vi "Insert Conditional.vi"(0 "Custom Type Test Executive in":refnum<class "Custom Type Test Executive.lvclass">, 1 "Name":string, 2 "Unique ID":string, 3 "Insertion Index":i32=-1, 4 "Assertion":refnum<class "Assert.lvclass">, 5 "error in (no error)":errorcluster, 6 "Parent ID":string, 7 "Variable X":string, 9 "Variable Y":string, 11 "Passing Executive":string, 13 "Failing Executive":string) -> (12 "Unique ID out":string, 14 "Custom Type Test Executive out":refnum<class "Custom Type Test Executive.lvclass">, 17 "Replaced?":bool, 19 "error out":errorcluster)   [LabVIEW 2017, in "Custom Type Test Executive.lvlib" / "Custom Type Test Executive.lvclass"]
uses:
  <vilib>/gpm_packages/@cs/test-executive/Source/Custom Type Test Executive/Custom Type Test Executive/Custom Type Test Executive.lvclass
  C:/Program Files/National Instruments/LabVIEW 2017/vi.lib/gpm_packages/@cs/test-executive/Source/Test Executive/TestExecutive/Test Executive.lvclass
  <vilib>/gpm_packages/@cs/run-time-assertions/Source/Assert/Assert.lvclass
  <vilib>/gpm_packages/@cs/test-executive/Source/Custom Type Test Executive/Conditional/Conditional.lvclass
  <vilib>/gpm_packages/@cs/data-type-serializer/source/Boolean/Boolean.lvclass/Boolean.ctl
  <vilib>/gpm_packages/@cs/test-executive/Source/Test Executive/TestExecutive/Test Executive.lvclass/Test Executive.ctl
  <vilib>/gpm_packages/@cs/data-type-serializer/source/Assertion/Assertion.lvclass/Assertion.ctl
  <vilib>/gpm_packages/@cs/data-type-serializer/source/String/String.lvclass/String.ctl
  ab7743c9-886f-4ba9-96ef-3eddb2be0c4c.vi
  3e0f2c71-549b-4a67-9684-e53ffa5485a3.vi
  d4ff8dc7-3c29-48bf-87c7-0a5f4c60658c.vi
  dd2f15b4-1a6c-43c8-9979-5ab3f4848fd4.vi
  23726e33-d18f-4018-bfd9-b10ab65a482d.vi
  439cc76c-a804-4d9c-815d-5f0c42b8a7d2.vi
  71fa445d-2d61-434e-a671-de836141d59d.vi
  <vilib>/gpm_packages/@cs/data-type-serializer/source/Assertion/Assertion.lvclass
  <vilib>/gpm_packages/@cs/data-type-serializer/source/String/String.lvclass
  <vilib>/gpm_packages/@cs/data-type-serializer/source/Boolean/Boolean.lvclass
  <vilib>/gpm_packages/@cs/linked-list/Source/Linked List/ILinkedList/ILinked List.lvclass
  <vilib>/gpm_packages/@cs/linked-list/Source/Linked List/Linked List Ref/Linked List Ref.lvclass
  <vilib>/gpm_packages/@cs/test-executive/Source/Test Executive/TestExecutive/Test Executive.lvclass
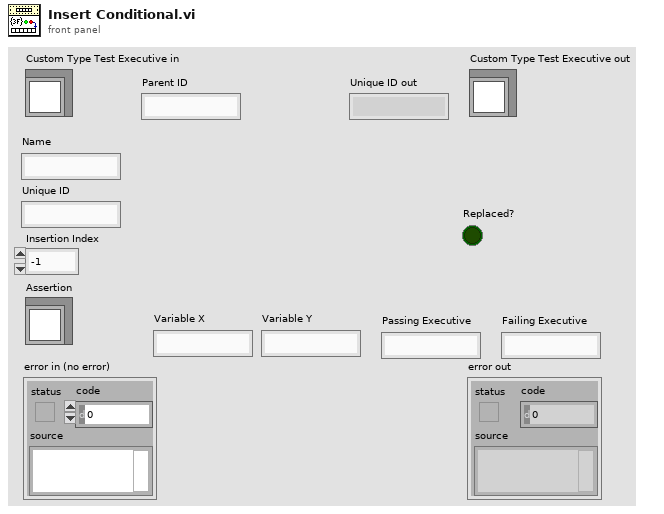
[diagram p1: front panel]
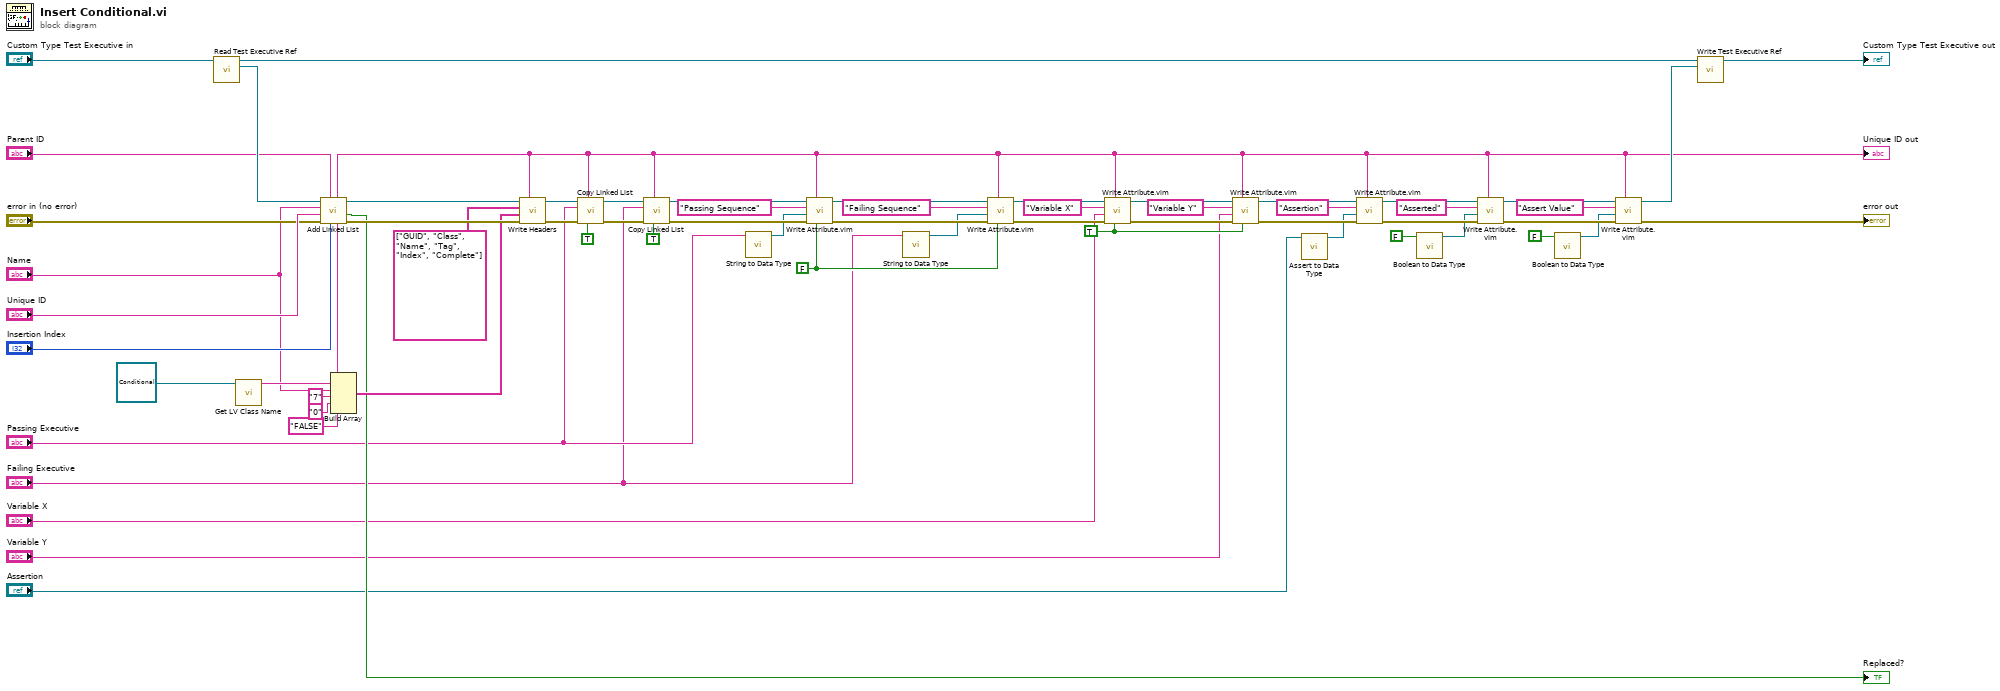
[diagram p0: block diagram]
diagram:
  w27 = FALSE ("Pointer?")
  w28 = TRUE ("Pointer?")
  n1 = call <vilib>:"Read Test Executive Ref.vi"("Test Executive in"="Custom Type Test Executive in") -> ("Test Executive Ref"=w25:refnum<data-value>, "Test Executive out"=w24:refnum<class "Custom Type Test Executive.lvclass">)  [unwired: 9 in]
  n2 = call <vilib>:"Get LV Class Name.vi"("object"=refnum<class "Conditional.lvclass"> refnum ("Custom Type Test Executive.lvlib:Conditional.lvclass")) -> ("class name"=w60:string)  [unwired: 9 in, 1 out]
  n3 = call <vilib>:"Add Linked List.vi"("Insertion Index"="Insertion Index", "Parent ID"="Parent ID", "error in (no error)"="error in (no error)", "Linked List ID"="Unique ID", "Name"="Name", "Linked List Ref"=w25) -> ("error out"=w62:errorcluster, "Replaced?"=→"Replaced?":bool, "Linked List Ref out"=w63:refnum<data-value>, "Linked List ID out"=w19:string)  [unwired: 2 in]
  "Unique ID out" <- w19
  n4 = Build Array(w19, w60, "Name", "7" ("element"), "0" ("element"), "FALSE" ("element")) -> (w58:string[])
  n5 = call <vilib>:"Write Headers.vi"("Linked List ID"=w19, "error in (no error)"=w62, "Header Values"=w58, "Header Names"=string[] ["GUID", "Class", "Name", "Tag", "Index", "Complete"], "Linked List Ref"=w63) -> ("error out"=w56:errorcluster, "Linked List Ref out"=w57:refnum<data-value>)  [unwired: 5 in]
  n6 = call <vilib>:"Copy Linked List.vi"("Move?"=TRUE, "New Parent Linked List ID"=w19, "error in (no error)"=w56, "Linked List ID"="Passing Executive", "Linked List Ref"=w57) -> ("error out"=w29:errorcluster, "Linked List Ref out"=w30:refnum<data-value>)  [unwired: 3 in, 2 out]
  n7 = call <vilib>:"Copy Linked List.vi"("Move?"=TRUE, "New Parent Linked List ID"=w19, "error in (no error)"=w29, "Linked List ID"="Failing Executive", "Linked List Ref"=w30) -> ("error out"=w54:errorcluster, "Linked List Ref out"=w55:refnum<data-value>)  [unwired: 3 in, 2 out]
  n8 = call <vilib>:"String to Data Type.vi"("String"="Passing Executive") -> ("Boolean out"=w9:refnum<class "String.lvclass">)  [unwired: 9 in, 1 out]
  n9 = call "Write Attribute.vim"("Pointer?"=w27, "Linked List ID"=w19, "error in (no error)"=w54, "Attribute"=w9, "Attribute Name"="Passing Sequence", "Linked List Ref"=w55) -> ("error out"=w51:errorcluster, "Linked List Ref out"=w52:refnum<data-value>)  [unwired: 2 in, 2 out]
  n10 = call <vilib>:"String to Data Type.vi"("String"="Failing Executive") -> ("Boolean out"=w7:refnum<class "String.lvclass">)  [unwired: 9 in, 1 out]
  n11 = call "Write Attribute.vim"("Pointer?"=w27, "Linked List ID"=w19, "error in (no error)"=w51, "Attribute"=w7, "Attribute Name"="Failing Sequence", "Linked List Ref"=w52) -> ("error out"=w47:errorcluster, "Linked List Ref out"=w49:refnum<data-value>)  [unwired: 2 in, 2 out]
  n12 = call "Write Attribute.vim"("Pointer?"=w28, "Linked List ID"=w19, "error in (no error)"=w47, "Attribute"="Variable X", "Attribute Name"="Variable X", "Linked List Ref"=w49) -> ("error out"=w45:errorcluster, "Linked List Ref out"=w46:refnum<data-value>)  [unwired: 2 in, 2 out]
  n13 = call "Write Attribute.vim"("Pointer?"=w28, "Linked List ID"=w19, "error in (no error)"=w45, "Attribute"="Variable Y", "Attribute Name"="Variable Y", "Linked List Ref"=w46) -> ("error out"=w42:errorcluster, "Linked List Ref out"=w43:refnum<data-value>)  [unwired: 2 in, 2 out]
  n14 = call <vilib>:"Assert to Data Type.vi"("Assert"="Assertion") -> ("Assert out"=w5:refnum<class "Assertion.lvclass">)  [unwired: 9 in, 1 out]
  n15 = call "Write Attribute.vim"("Linked List ID"=w19, "error in (no error)"=w42, "Attribute"=w5, "Attribute Name"="Assertion", "Linked List Ref"=w43) -> ("error out"=w39:errorcluster, "Linked List Ref out"=w40:refnum<data-value>)  [unwired: 3 in, 2 out]
  n16 = call <vilib>:"Boolean to Data Type.vi"("Boolean"=FALSE) -> ("Boolean out"=w3:refnum<class "Boolean.lvclass">)  [unwired: 9 in, 1 out]
  n17 = call "Write Attribute.vim"("Linked List ID"=w19, "error in (no error)"=w39, "Attribute"=w3, "Attribute Name"="Asserted", "Linked List Ref"=w40) -> ("error out"=w36:errorcluster, "Linked List Ref out"=w37:refnum<data-value>)  [unwired: 3 in, 2 out]
  n18 = call <vilib>:"Boolean to Data Type.vi"("Boolean"=FALSE) -> ("Boolean out"=w1:refnum<class "Boolean.lvclass">)  [unwired: 9 in, 1 out]
  n19 = call "Write Attribute.vim"("Linked List ID"=w19, "error in (no error)"=w36, "Attribute"=w1, "Attribute Name"="Assert Value", "Linked List Ref"=w37) -> ("error out"=→"error out":errorcluster, "Linked List Ref out"=w22:refnum<data-value>)  [unwired: 3 in, 2 out]
  n20 = call <vilib>:"Write Test Executive Ref.vi"("Test Executive Ref"=w22, "Test Executive in"=w24) -> ("Test Executive out"=→"Custom Type Test Executive out":refnum<class "Custom Type Test Executive.lvclass">)  [unwired: 9 in]
